vi "subvi for voltech.vi"(7 "Measurement Results 2":string[][](array[string])) -> (1 "Array":string[](array[string]))   [LabVIEW 2011]
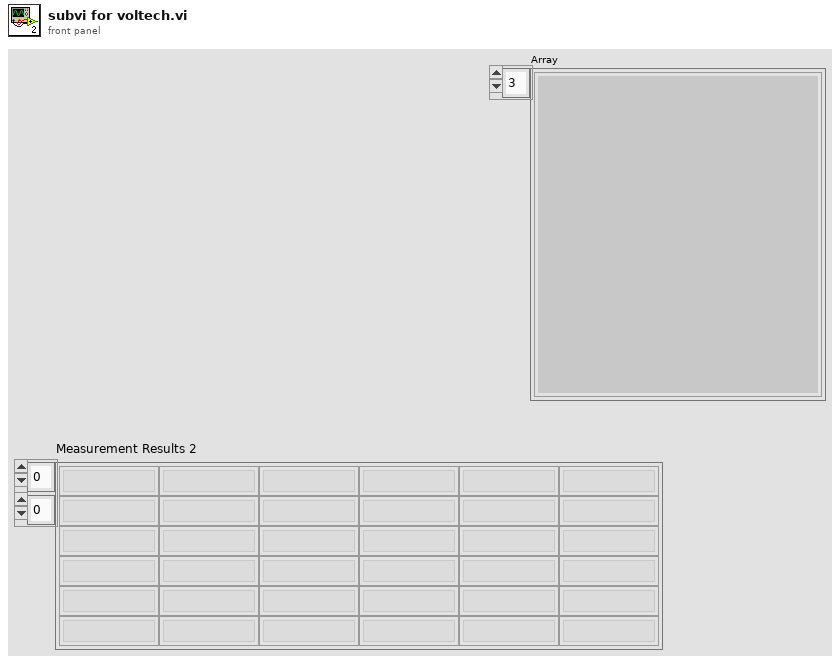
[diagram p1: front panel]
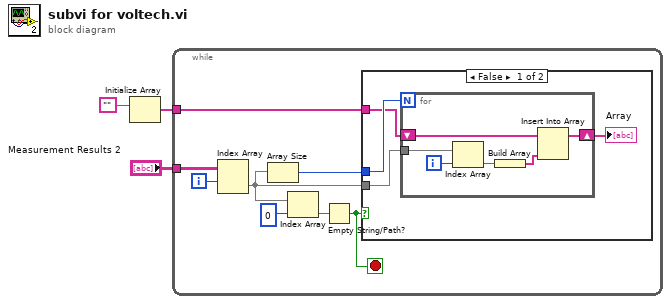
[diagram p0: block diagram]
diagram:
  n1 = Initialize Array("") -> (w2:string[])  [unwired: 1 in]
  n2 = while {
    tunnel: w2 -> [w6]
    tunnel: "Measurement Results 2" -> [w5]
    i -> [w11]
    stop <- w4 stop-if-true
    n3 = Index Array(array=w5, index (row)=w11) -> (element=w7:string[])  [unwired: 1 in]
    n4 = Array Size(array=w7) -> (size(s)=w8:i32)
    n5 = Index Array(array=w7, index=0) -> (element=w9:string)
    n6 = Empty String/Path?(string/path=w9) -> (empty?=w4:bool)
    n7 = case shown="False" w4 {
      tunnel: w8 -> [w15 _]
      tunnel: w7 -> [w14 _]
      tunnel: w6 -> [w13 _]
      frame False {
        n8 = for {
          N: w15 -> [_]
          tunnel: w14 -> [w21]
          shift-right: [w17] -> w12
          shift-left: w13 -> [w18]
          i -> [w20]
          n9 = Index Array(array=w21, index=w20) -> (element=w16:string)
          n10 = Build Array(w16) -> (w19:string[])
          n11 = Insert Into Array(array=w18, new element=w19) -> (w17:string[])  [unwired: 1 in]
        }
        "Array" <- w12
      }
      frame True {
      }
    }
  }
